vi "Read Element of Tags.vi"(10 "index":i32, 11 "Series in":refnum<class "Series.lvclass">) -> (2 "TagSet":T1, 3 "Series out":refnum<class "Series.lvclass">)   [LabVIEW 2018, in "InfluxDB Client.lvlib" / "Series.lvclass"]
uses:
  Series.lvclass
  Controls/TagSet.ctl
  Series.lvclass/Series.ctl
  InfluxDB Client.lvlib
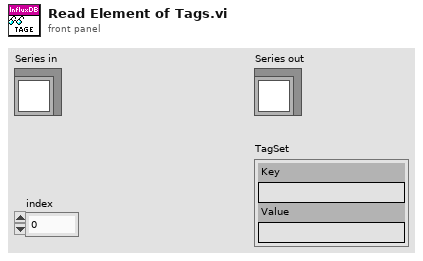
[diagram p1: front panel]
types:
  T1 = typedef "InfluxDB Client.lvlib/TagSet.ctl" = cluster{"Key":string, "Value":string}
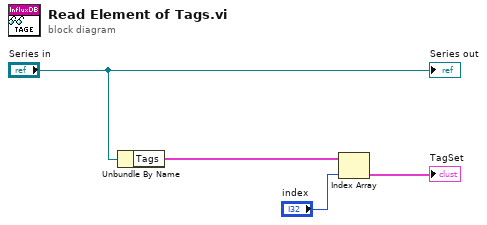
[diagram p0: block diagram]
diagram:
  n1 = Unbundle By Name("Series in") -> ("Tags"=w2:T1[])
  n2 = Index Array(array=w2, index="index") -> (element=→"TagSet":T1)
  "Series out" <- "Series in"
